vi "Open Log File .vi"(4 "File Name Snippet":string, 5 "Log Path":path) -> (1 "appended path":path, 2 "Byte Stream File out":refnum<file>)   [LabVIEW 2019]
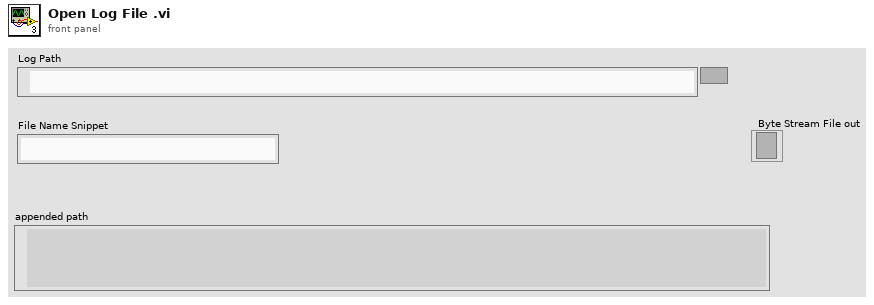
[diagram p1: front panel]
types:
  T1 = enum16{"open", "replace", "create", "open or create", "replace or create", "replace or create with confirmation"}
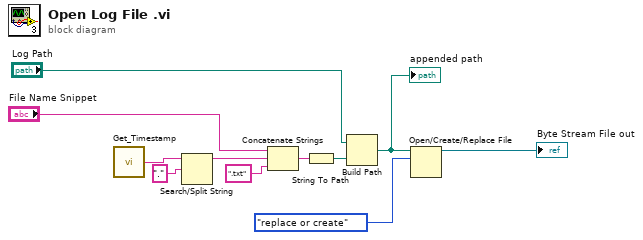
[diagram p0: block diagram]
diagram:
  n1 = call "Get_Timestamp.vi"() -> ("date/time string"=w11:string)  [unwired: 1 in]
  n2 = Search/Split String(string=w11, search string/char (-)=".") -> (substring before match=w9:string)  [unwired: 1 in, 2 out]
  n3 = Concatenate Strings("File Name Snippet", w9, ".txt" ("string")) -> (w6:string)
  n4 = String To Path(string=w6) -> (path=w5:path)
  n5 = Build Path(base path="Log Path", name or relative path=w5) -> (appended path=w3:path)
  "appended path" <- w3
  n6 = Open/Create/Replace File(file path (use dialog)=w3, operation (0:open)=T1."replace or create") -> (refnum out=→"Byte Stream File out":refnum<file>)  [unwired: 4 in, 2 out]
